vi "Calculate Extraction Rect.vi"(11 "Particle Rect":T1) -> (3 "Test Rect":dbl[](array[numeric]))   [LabVIEW 2025]
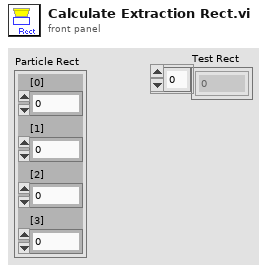
[diagram p1: front panel]
types:
  T1 = cluster{"[0]":dbl, "[1]":dbl, "[2]":dbl, "[3]":dbl}
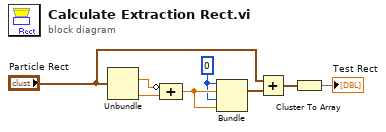
[diagram p0: block diagram]
diagram:
  w4 = 0
  n1 = Unbundle("Particle Rect") -> ("[1]"=w7:dbl, "[3]"=w6:dbl)  [unwired: 2 out]
  n2 = Compound Arithmetic op=ADD(invert w7, w6) -> (w5:dbl)
  n3 = Bundle(w4, w5, w4, w5) -> (w3:cluster{i32, dbl, i32, dbl})  [unwired: 1 in]
  n4 = Add(x="Particle Rect", y=w3) -> (x+y=w2:cluster{dbl, dbl, dbl, dbl})
  n5 = Cluster To Array(cluster=w2) -> (array=→"Test Rect":dbl[])
